vi "CMD Append String To Log.vi"(8 "error in (no error)":errorcluster, 10 "StringToAppend":string, 11 "LogEngine in":refnum<class "LogEngine.lvclass">) -> (0 "error out":errorcluster, 3 "LogEngine out":refnum<class "LogEngine.lvclass">)   [LabVIEW 2017, in "LogEngine.lvclass"]
doc: "Developed by Kevin Thompson\nkevin@thompsonengineering.net\n\nCopyright 2018-2020\nThompson Engineering, LLC"
uses:
  LogEngine.lvclass
  Data Types/AsyncCmd_LogEngine--enum.ctl
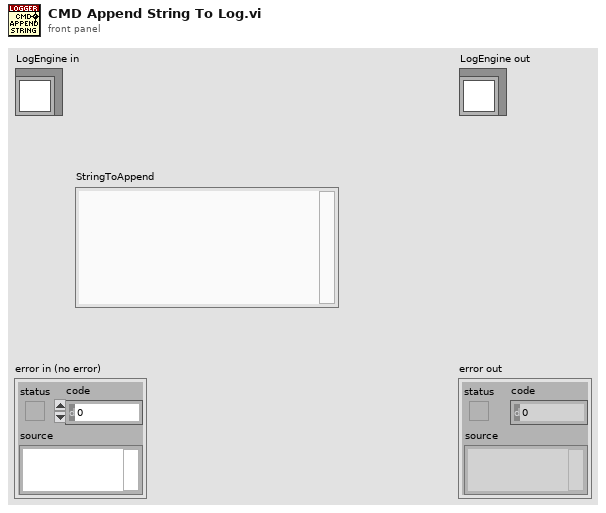
[diagram p1: front panel]
types:
  T1 = typedef "LogEngine.lvclass/AsyncCmd_LogEngine--enum.ctl" = enum16{"LE.CreateLogFile", "LE.EnableLogging", "LE.OpenTDMS", "LE.CloseTDMS", "LE.StartTDMSLogging", "LE.StopTDMSLogging", "LE.AppendStrToLog"}
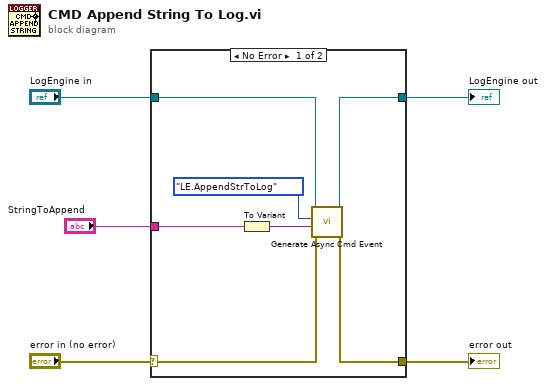
[diagram p0: block diagram]
diagram:
  n1 = case shown="No Error" "error in (no error)" {
    selector: "error in (no error)" -> [w10 w14]
    tunnel: [w9 w14] -> w4
    tunnel: [w11 w13] -> w2
    tunnel: "LogEngine in" -> [w12 w13]
    tunnel: "StringToAppend" -> [w7 _]
    frame No Error {
      n2 = To Variant(anything=w7) -> (Variant=w6:variant)
      n3 = call "Generate Async Cmd Event.vi"("error in (no error)"=w10, "vData"=w6, "AsyncCmd"=AsyncCmd_LogEngine--enum."LE.AppendStrToLog", "LogEngine"=w12) -> ("error out"=w9:errorcluster, "LogEngine out"=w11:refnum<class "LogEngine.lvclass">)  [unwired: 6 in]
    }
    frame Error {
    }
  }
  "error out" <- w4
  "LogEngine out" <- w2
